vi "tt20_get_correlation.vi"(8 "error in (no error)":errorcluster, 11 "tt20 in":refnum<class "tt20.lvclass">) -> (0 "error out":errorcluster, 2 "histogram":cluster{dbl[], dbl[]}[](array[cluster]), 3 "tt20 out":refnum<class "tt20.lvclass">)   [LabVIEW 2015, in "tt20.lvclass"]
uses:
  tt20.lvclass
  tt20.lvclass/tt20.ctl
  C:/Users/MX-Microscope/Documents/LabVIEW Data/lvoop_campus_2018/Detector_Class/Swabian/time_tagger_vis/TTCSharp32.dll
  time_tagger_vis/TTCSharp32.dll
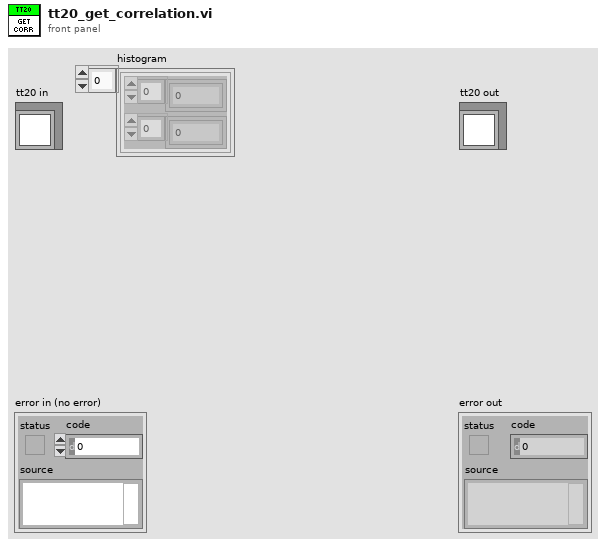
[diagram p1: front panel]
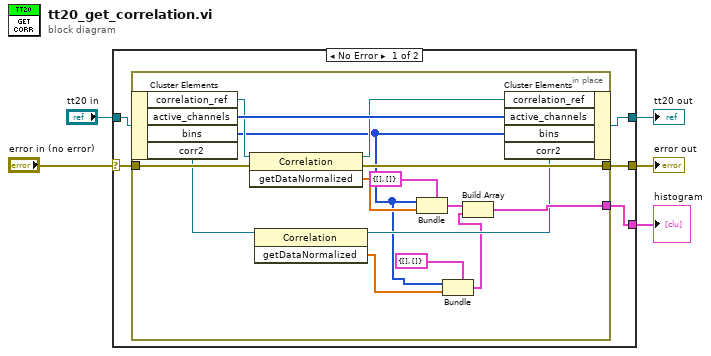
[diagram p0: block diagram]
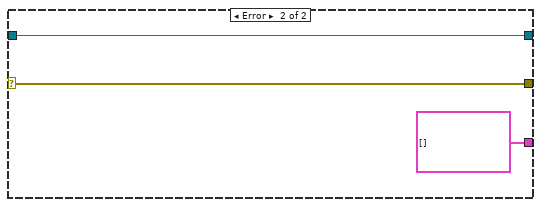
[diagram p2: hidden frame]
diagram:
  n1 = case shown="No Error" "error in (no error)" {
    selector: "error in (no error)" -> [w9 w28]
    tunnel: "tt20 in" -> [w10 w27]
    tunnel: [w8 w27] -> w3
    tunnel: [w7 w28] -> w2
    tunnel: [w6 cluster{dbl[], dbl[]}[] []] -> w1
    frame No Error {
      n2 = in-place {
        in-place-border: w9 -> [w22]
        in-place-border: [w21] -> w7
        in-place-border: [w17] -> w6
        n3 = in-place-cluster #1(w10) -> ("correlation_ref"=w24:refnum<k24>, "active_channels"=w25:u32[], "bins"=w12:i64[], "corr2"=w16:refnum<k24>)
        n4 = invoke class="Correlation" method="getDataNormalized"(reference=w24, error in=w22) -> (reference out=w23:refnum<k24>, error out=w21:errorcluster, "getDataNormalized"=w20:dbl[])  [unwired: 1 in]
        n5 = invoke class="Correlation" method="getDataNormalized"(reference=w16) -> (reference out=w15:refnum<k24>, "getDataNormalized"=w13:dbl[])  [unwired: 2 in, 1 out]
        n6 = Bundle(cluster=cluster{dbl[], dbl[]} {[], []} ("element"), w12, w20) -> (w18:cluster{dbl[], dbl[]})
        n7 = Bundle(cluster=cluster{dbl[], dbl[]} {[], []} ("element"), w12, w13) -> (w11:cluster{dbl[], dbl[]})
        n8 = Build Array(w18, w11) -> (w17:cluster{dbl[], dbl[]}[])
        n9 = in-place-cluster #1("correlation_ref"=w23, "active_channels"=w25, "bins"=w12, "corr2"=w15) -> (w8:refnum<class "tt20.lvclass">)
      }
    }
    frame Error {
    }
  }
  "error out" <- w2
  "tt20 out" <- w3
  "histogram" <- w1
